vi "Read Temperature Curve from File.vi"(8 "error in (no error)":errorcluster, 11 "KIT-QA in":refnum<class "KIT-QA.lvclass">) -> (0 "error out":errorcluster, 3 "KIT-QA out":refnum<class "KIT-QA.lvclass">)   [LabVIEW 2015, in "KIT-QA.lvlib" / "KIT-QA.lvclass"]
doc: "Reads out the temperature data provided by KIT-IntegralCalibration from file as specified."
uses:
  KIT-QA.lvclass
  <vilib>/Utility/file.llb/Read Delimited Spreadsheet (string).vi
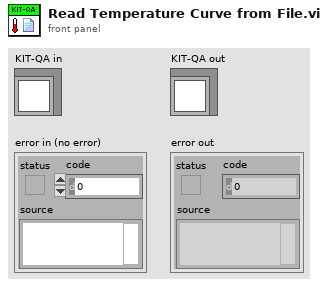
[diagram p1: front panel]
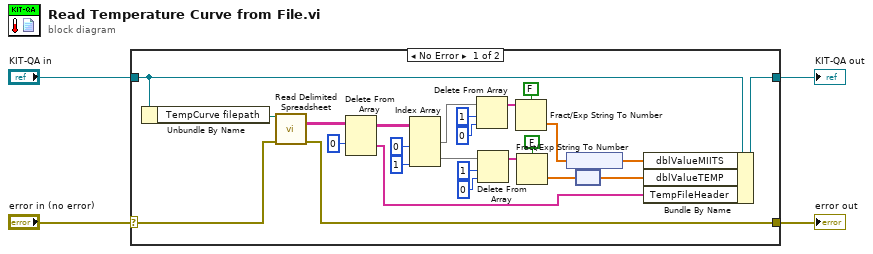
[diagram p0: block diagram]
diagram:
  n1 = case shown="No Error" "error in (no error)" {
    selector: "error in (no error)" -> [w8 w31]
    tunnel: [w7 w31] -> w3
    tunnel: [w25 w30] -> w1
    tunnel: "KIT-QA in" -> [w26 w30]
    frame No Error {
      n2 = Unbundle By Name(w26) -> ("TempCurve filepath"=w28:path)
      n3 = call-poly <vilib>:"Read Delimited Spreadsheet.vi"("file path (dialog if empty)"=w28, "error in (no error)"=w8) -> ("all rows"=w27:string[][], "error out"=w7:errorcluster)  [unwired: 8 in, 4 out]
      n4 = Delete From Array(array=w27, index (row)=0) -> (deleted portion=w11:string[], array with subset deleted=w12:string[][])  [unwired: 2 in]
      n5 = Index Array(array=w12, index (col) #1=0 ("disabled index (col)"), index (col) #2=1 ("index (col)")) -> (element #1=w22:string[], element #2=w21:string[])  [unwired: 2 in]
      n6 = Delete From Array(array=w22, length=1, index=0) -> (array with subset deleted=w17:string[])  [unwired: 1 out]
      n7 = Delete From Array(array=w21, length=1, index=0) -> (array with subset deleted=w18:string[])  [unwired: 1 out]
      n8 = Fract/Exp String To Number(use system decimal point (T)=FALSE, string=w17) -> (number=w10:dbl[])  [unwired: 2 in, 1 out]
      n9 = Fract/Exp String To Number(use system decimal point (T)=FALSE, string=w18) -> (number=w9:dbl[])  [unwired: 2 in, 1 out]
      n10 = node(w10) -> (w5:dbl[unit][])
      n11 = node(w9) -> (w6:dbl[unit][])
      n12 = Bundle By Name(cluster=w26, "dblValueMIITS"=w5, "dblValueTEMP"=w6, "TempFileHeader"=w11) -> (w25:refnum<class "KIT-QA.lvclass">)
    }
    frame Error {
    }
  }
  "error out" <- w3
  "KIT-QA out" <- w1
